vi "Benchmark Convert String Type - Single Type to Single Type.vi"(5 "src data type":T1, 7 "dst data type":T1, 8 "iterations (1)":i32=1, 9 "dst byte order":T2(ring)=enum."native, host order", 10 "src byte order":T2(ring), 11 "channel count":i32=10000 format="%#.3p") -> (0 "error out":errorcluster, 3 "duration":dbl format="%.0ps")   [LabVIEW 2017]
uses:
  Typedefs/DSF Data Type.ctl
  Classes/Buffer Converter/Convert String Type Subset.vi
  VIs/Sizeof 1D.vi
  VIs/Sizeof.vi
  Classes/Buffer Converter/Buffer Converter.lvclass
  DSF Core.lvlib
panel:
  out "dst buffer size":u64 format="%.0pB"
  out "src buffer size":u64 format="%.0pB"
  out "src buffer":string
  out "dst buffer":string
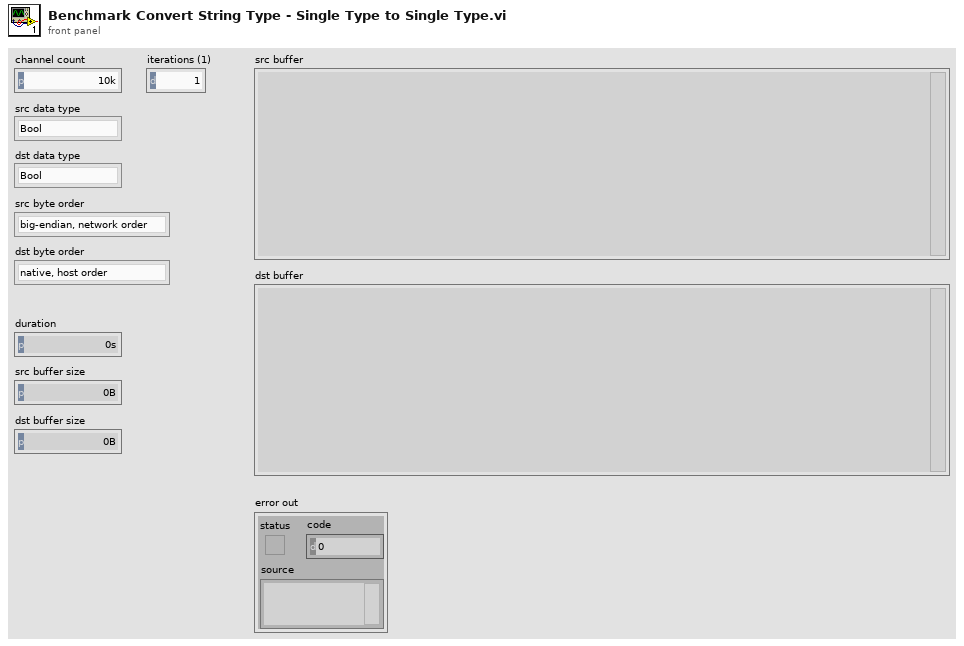
[diagram p1: front panel]
types:
  T1 = typedef "DSF Core.lvlib/DSF Data Type.ctl" = enum8{"Bool", "SGL", "DBL", "I8", "I16", "I32", "I64", "U8", "U16", "U32", "U64"}
  T2 = enum16{"big-endian, network order", "native, host order", "little-endian"}
  T3 = typedef "DSF Core.lvlib/Buffer Converter.lvclass/Type Conversion.ctl" = cluster{"unconverted descriptor":T4, "converted descriptor":T4, "channel count":u64}
  T4 = typedef "DSF Core.lvlib/Buffer.lvclass/Channel Descriptor.ctl" = cluster{"buffer offset":u64, "data type":T1}
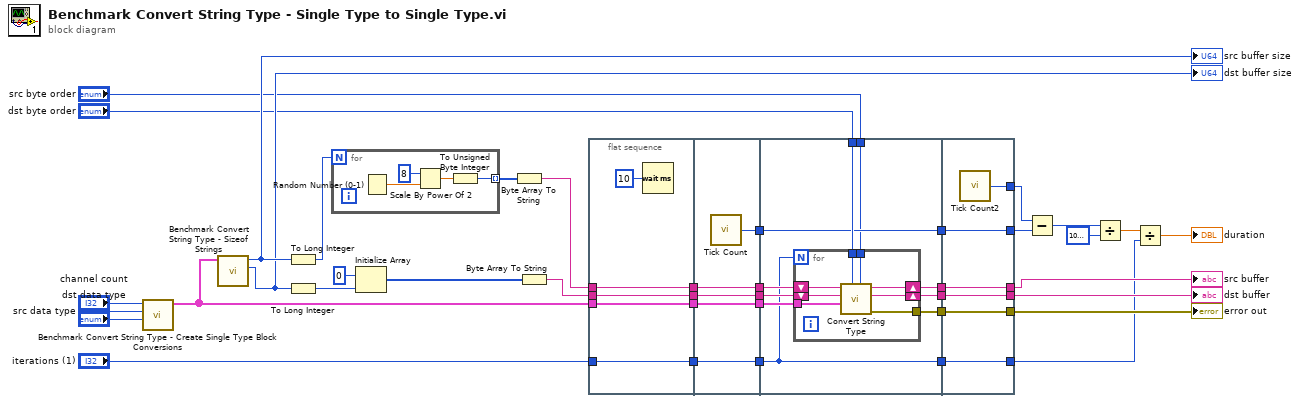
[diagram p0: block diagram]
diagram:
  n1 = call "Benchmark Convert String Type - Create Single Type Block Conversions.vi"("dst data type"="dst data type", "src data type"="src data type", "channel count"="channel count") -> ("conversions"=w40:T3[])  [unwired: 8 in]
  n2 = call "Benchmark Convert String Type - Sizeof Strings.vi"("conversions"=w40) -> ("converted string size"=w37:u64, "unconverted string size"=w39:u64)  [unwired: 9 in]
  "src buffer size" <- w39
  "dst buffer size" <- w37
  n3 = To Long Integer(number=w39) -> (32bit integer=w13:i32)
  n4 = To Long Integer(number=w37) -> (32bit integer=w36:i32)
  n5 = for {
    N: w13 -> [_]
    tunnel: [w41] -> w12 mode=indexing
    n6 = Random Number (0-1)() -> (number: 0 to 1=w43:dbl)
    n7 = Scale By Power Of 2(n=i16 8, x=w43) -> (x*2^n=w42:dbl)
    n8 = To Unsigned Byte Integer(number=w42) -> (unsigned 8bit integer=w41:u8)
  }
  n9 = Initialize Array(u8 0 ("element"), w36) -> (w35:u8[])
  n10 = Byte Array To String(unsigned byte array=w12) -> (string=w34:string)
  n11 = Byte Array To String(unsigned byte array=w35) -> (string=w11:string)
  n12 = flat-sequence {
    tunnel: w34 -> [w47]
    tunnel: w11 -> [w48]
    tunnel: w40 -> [w49]
    tunnel: [w49] -> w22
    tunnel: [w48] -> w21
    tunnel: [w47] -> w20
    tunnel: "iterations (1)" -> [w45]
    tunnel: [w45] -> w6
    tunnel: [w54] -> w25
    tunnel: [w53] -> w24
    tunnel: [w52] -> w23
    tunnel: w22 -> [w54]
    tunnel: w21 -> [w53]
    tunnel: w20 -> [w52]
    tunnel: [w51] -> w19
    tunnel: w6 -> [w50]
    tunnel: [w50] -> w5
    tunnel: "dst byte order" -> [w58]
    tunnel: "src byte order" -> [w56]
    tunnel: [w59] -> w28
    tunnel: [w60] -> w27
    tunnel: [w61] -> w26
    tunnel: w25 -> [w64]
    tunnel: w24 -> [w63]
    tunnel: w23 -> [w62]
    tunnel: w19 -> [w57]
    tunnel: [w57] -> w18
    tunnel: w5 -> [w55]
    tunnel: [w55] -> w4
    tunnel: [w76] -> w30
    tunnel: [w77] -> w31
    tunnel: [w78] -> w32
    tunnel: w28 -> [w78]
    tunnel: w27 -> [w77]
    tunnel: w26 -> [w76]
    tunnel: [w75] -> w16
    tunnel: w18 -> [w74]
    tunnel: [w74] -> w17
    tunnel: w4 -> [w73]
    tunnel: [w73] -> w2
    frame #0 {
      n13 = Wait (ms)(milliseconds to wait=u32 10) -> ()  [unwired: 1 out]
    }
    frame #1 {
      n14 = call "Tick Count"() -> ("Tick Count(uSec)"=w51:u32)
    }
    frame #2 {
      n15 = for {
        N: w55 -> [_]
        tunnel: w64 -> [w72]
        tunnel: w58 -> [w69]
        tunnel: w56 -> [w68]
        tunnel: [w67] -> w59
        shift-right: [w66] -> w60
        shift-left: w63 -> [w71]
        shift-right: [w65] -> w61
        shift-left: w62 -> [w70]
        n16 = call "Convert String Type.vi"("src byte order"=w68, "dst byte order"=w69, "conversions"=w72, "dst buffer in"=w71, "src buffer in"=w70) -> ("error out"=w67:errorcluster, "dst buffer out"=w66:string, "src buffer out"=w65:string)  [unwired: 4 in]
      }
    }
    frame #3 {
      n17 = call "Tick Count2"() -> ("Tick Count(uSec)"=w75:u32)
    }
  }
  n18 = Subtract(x=w16, y=w17) -> (x-y=w15:u32)
  n19 = Divide(x=w15, y=u32 1000000) -> (x/y=w3:dbl)
  n20 = Divide(x=w3, y=w2) -> (x/y=→"duration":dbl)
  "error out" <- w32
  "dst buffer" <- w31
  "src buffer" <- w30
